vi "MaxStatus.vi"(0 "VisaCluster":T2, 11 "error in (no error)":errorcluster) -> (4 "VisaCluster":T2, 8 "Answer":string, 10 "Max":T1, 15 "error out":errorcluster)   [LabVIEW 2014, in "FH 55.lvlib"]
doc: "Dieses VI gibt den Status der Extremwertausgabe zurück. Die möglichen Ausgaben sind:\n keine Extermwertausgabe \n nur Max-Werte\n Max und Min-Werte\n\nThis VI returns the status of extreme value output. The possible issues are:\n no extreme value output\n only Max values\n Max and Min values"
uses:
  FH 55.lvlib
  TypeDef/VisaCluster.ctl
  TypeDef/Max.ctl
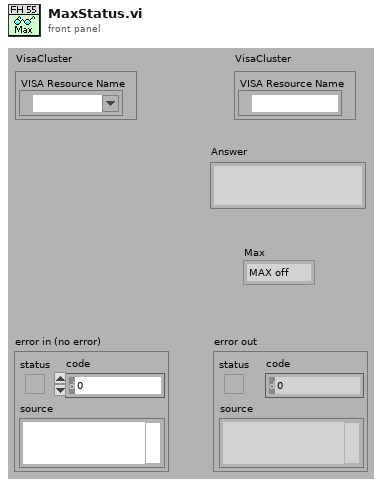
[diagram p1: front panel]
types:
  T1 = typedef "FH 55.lvlib/Max.ctl" = enum16{"MAX off", "Show MAX", "MAX/MIN"}
  T2 = typedef "FH 55.lvlib/VisaCluster.ctl" = cluster{"VISA Resource Name":refnum<visa-resource-name>}
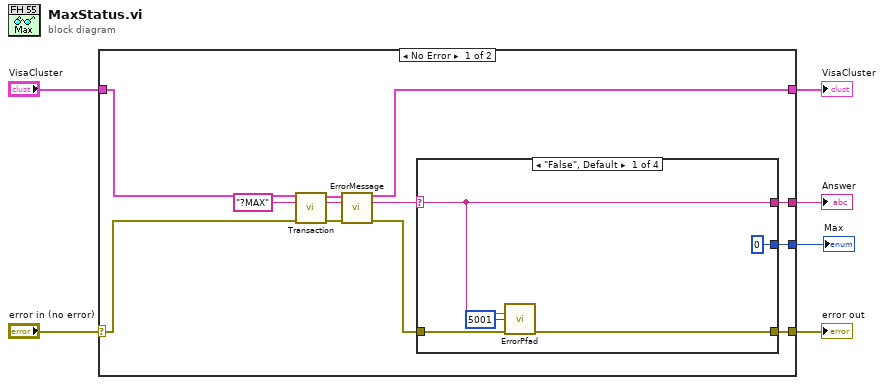
[diagram p0: block diagram]
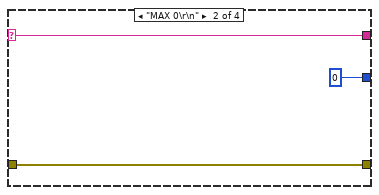
[diagram p2: hidden frame]
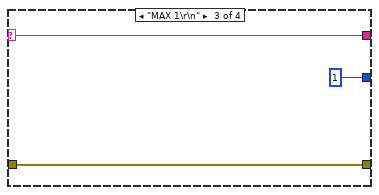
[diagram p3: hidden frame]
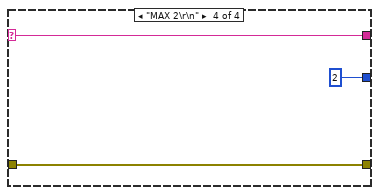
[diagram p4: hidden frame]
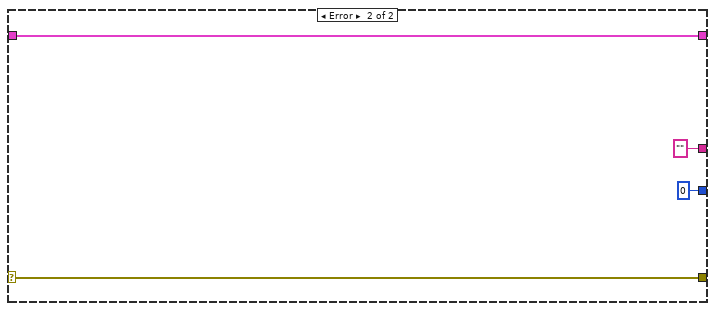
[diagram p5: hidden frame]
diagram:
  n1 = case shown="No Error" "error in (no error)" {
    selector: "error in (no error)" -> [w7 w35]
    tunnel: "VisaCluster" -> [w8 w36]
    tunnel: [w18 w36] -> w2
    tunnel: [w13 w35] -> w4
    tunnel: [w12 ""] -> w3
    tunnel: [w9 0] -> w1
    frame No Error {
      n2 = call "Transaction.vi"("VisaCluster"=w8, "Command"="?MAX", "error in (no error)"=w7) -> ("VisaCluster"=w16:T2, "Answer"=w11:string, "error out"=w17:errorcluster)  [unwired: 9 in, 1 out]
      n3 = call "ErrorMessage.vi"("VisaCluster"=w16, "Message In"=w11, "error in (no error)"=w17) -> ("VisaCluster"=w18:T2, "Message Out"=w10:string, "error out"=w14:errorcluster)  [unwired: 10 in]
      n4 = case shown="\"False\", Default" w10 {
        selector: w10 -> [w20 w26 w29 w32]
        tunnel: w14 -> [w22 w25 w28 w31]
        tunnel: [w21 w25 w28 w31] -> w13
        tunnel: [w20 w26 w29 w32] -> w12
        tunnel: [0 0 1 2] -> w9
        frame "False", Default {
          n5 = call "ErrorPfad.vi"("Message In"=w20, "Numeric"=5001, "error in (no error)"=w22) -> ("error out"=w21:errorcluster)  [unwired: 11 in, 1 out]
        }
        frame "MAX 0\r\n" {
        }
        frame "MAX 1\r\n" {
        }
        frame "MAX 2\r\n" {
        }
      }
    }
    frame Error {
    }
  }
  "error out" <- w4
  "Answer" <- w3
  "VisaCluster" <- w2
  "Max" <- w1
